vi "list name ROI.vi"(6 "debug?":bool, 8 "error in":errorcluster, 11 "Elements Selected":string[][](array[string])=[["0.000000", "1.951680", "Ca", "Escape Peak"], ["1.000000", "2.30784", "S", "Ka1"], ["2.000000", "2.62239", "Cl", "Ka1"], ["3.000000", "2.9577", "Ar", "Ka1"], ["4.000000", "3.3138", "K", "Ka1"], ["5.000000", "3.69168", "Ca", "Ka1"], ["6.000000", "4.0127", "Ca", "Kb1"], ["7.000000", "4.51084", "Ti", "Ka1"], ["8.000000", "5.89875", "Mn", "Ka1"], ["9.000000", "6.40384", "Fe", "Ka1"], ["10.000000", "7.05798", "Fe", "Kb1"], ["11.000000", "8.04778", "Cu", "Ka1"], ["12.000000", "8.63886", "Zn", "Ka1"]]) -> (0 "error out":errorcluster, 3 "ROIs List":cluster{"String":string, "Value":i32}[](array[cluster]))   [LabVIEW 2023]
uses:
  <vilib>/Utility/miscctls.llb/LVStringsAndValuesArrayTypeDef_U16.ctl
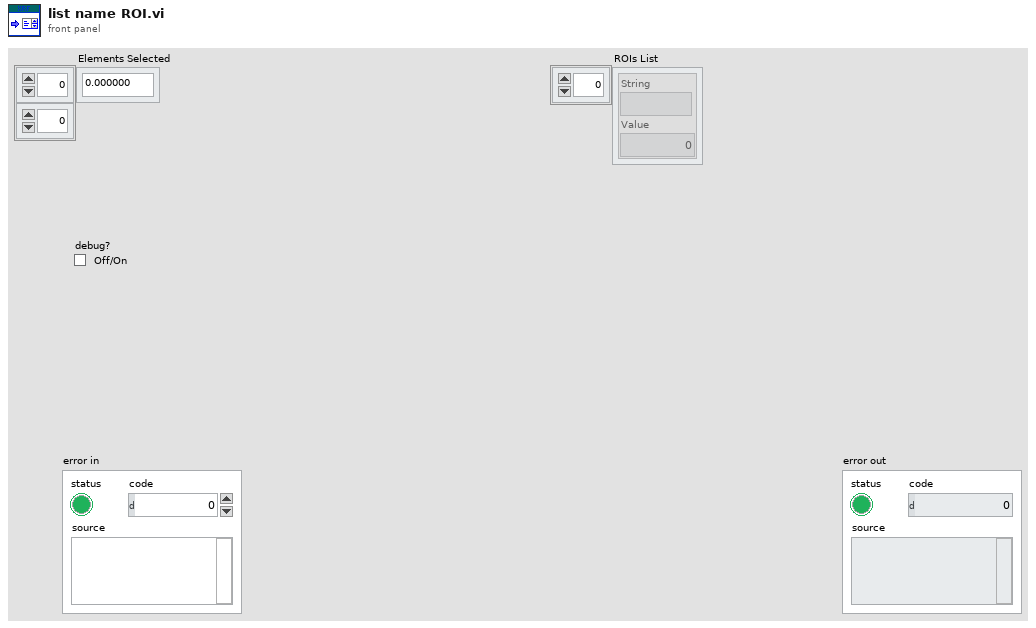
[diagram p1: front panel]
types:
  T1 = typedef "LVStringsAndValuesArrayTypeDef_U16.ctl" = cluster{"String":string, "Value":u16}[]
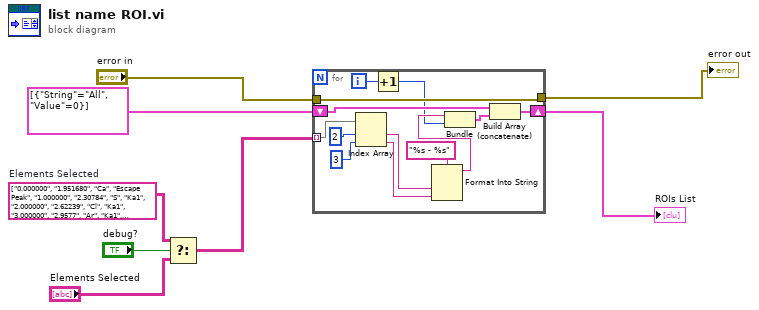
[diagram p0: block diagram]
diagram:
  w5 = string[][] [["0.000000", "1.951680", "Ca", "Escape Peak"], ["1.000000", "2.30784", "S", "Ka1"], ["2.000000", "2.62239", "Cl", "Ka1"], ["3.000000", "2.9577", "Ar", "Ka1"], ["4.000000", "3.3138", "K", "Ka1"], ["5.000000", "3.69168", "Ca", "Ka1"], ["6.000000", "4.0127", "Ca", "Kb1"], ["7.000000", "4.51084", "Ti", "Ka1"], ["8.000000", "5.89875", "Mn", "Ka1"], ["9.000000", "6.40384", "Fe", "Ka1"], ["10.000000", "7.05798", "Fe", "Kb1"], ["11.000000", "8.04778", "Cu", "Ka1"], ["12.000000", "8.63886", "Zn", "Ka1"]]  # Elements Selected
  n1 = Select(t=w5, s="debug?", f="Elements Selected") -> (s? t:f=w3:string[][])
  n2 = for {
    tunnel: w3 -> [w17] mode=indexing
    shift-right: [w20] -> w1
    shift-left: T1 [{"String"="All", "Value"=0}] ("Strings And Values []") -> [w19]
    tunnel: "error in" -> [w15]
    tunnel: [w15] -> w2
    i -> [w18]
    n3 = Index Array(array=w17, index #1=2 ("index"), index #2=3 ("index")) -> (element #1=w12:string, element #2=w11:string)
    n4 = Increment(x=w18) -> (x+1=w9:i32)
    n5 = Format Into String(format string="%s - %s", w12, w11) -> (resulting string=w10:string)  [unwired: 2 in, 1 out]
    n6 = Bundle(w10, w9) -> (w21:cluster{string, i32})  [unwired: 1 in]
    n7 = Build Array (concatenate)(w19, w21) -> (w20:cluster{"String":string, "Value":i32}[])
  }
  "error out" <- w2
  "ROIs List" <- w1
